vi "Write ExportSignal.vi"(8 "error in (no error)":errorcluster, 10 "Export Signal":T1={"signal"=12487, "Destination"="/PXI1Slot6/PFI3", "Route"="/PXI1Slot6/PXI_Trig5"} {"signal" items=["AI Convert Clock"=12484, "10MHz Reference Clock"=12536, "20MHz Timebase Clock"=12486, "Sample Clock"=12487, "Advance Trigger"=12488, "Reference Trigger"=12490, "Start Trigger"=12491, "Advance Complete Event"=12492, "AI Hold Complete Event"=12493, "Counter Output Event"=12494, "Change Detection Event"=12511, "Watchdog Timer Expired Event"=12512]}, 11 "NiPxi6733 in":refnum<class "NiPxi6733.lvclass">) -> (0 "error out":errorcluster, 3 "NiPxi6733 out":refnum<class "NiPxi6733.lvclass">)   [LabVIEW 2018, in "FgenPlugins.lvlib" / "NiPxi6733.lvclass"]
uses:
  NiPxi6733.lvclass
  Typedefs/ExportSignal.ctl
  NiPxi6733.lvclass/NiPxi6733.ctl
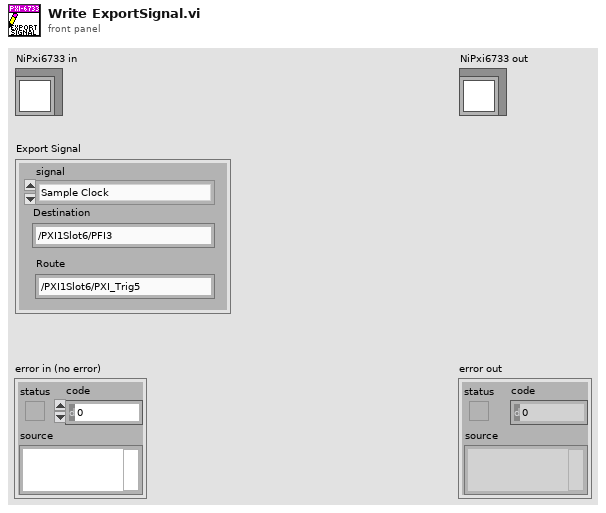
[diagram p1: front panel]
types:
  T1 = typedef "FgenPlugins.lvlib/NiPxi6733.lvclass/ExportSignal.ctl" = cluster{"signal":i32, "Destination":string, "Route":string}
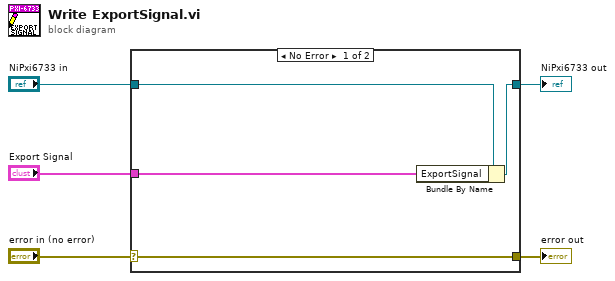
[diagram p0: block diagram]
diagram:
  n1 = case shown="No Error" "error in (no error)" {
    selector: "error in (no error)" -> [w9 w10]
    tunnel: [w9 w10] -> w4
    tunnel: [w7 w11] -> w2
    tunnel: "NiPxi6733 in" -> [w8 w11]
    tunnel: "Export Signal" -> [w6 _]
    frame No Error {
      n2 = Bundle By Name(cluster=w8, "ExportSignal"=w6) -> (w7:refnum<class "NiPxi6733.lvclass">)
    }
    frame Error {
    }
  }
  "error out" <- w4
  "NiPxi6733 out" <- w2
